vi "portOpen.vi"(3 "COMport":string="COM6") -> (0 "error out":errorcluster)   [LabVIEW 2015]
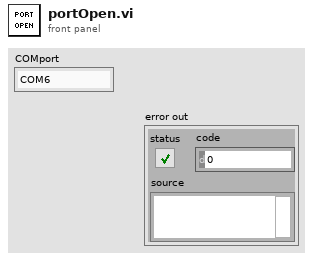
[diagram p1: front panel]
types:
  T1 = cluster{"OpenPort":bool, "ClosePort":bool, "Baudrate":i32, "Wait":u16, "ReadWrite":bool}
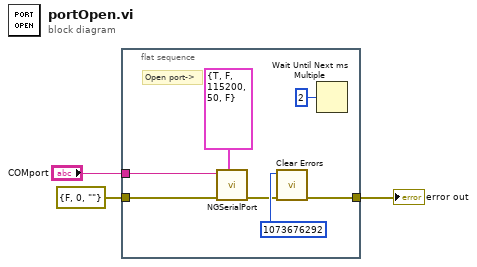
[diagram p0: block diagram]
diagram:
  n1 = flat-sequence {
    tunnel: "COMport" -> [w10]
    tunnel: [w8] -> w2
    tunnel: errorcluster {"status"=FALSE, "code"=0, "source"=""} ("error in") -> [w6]
    frame #0 {
      # "Open port->"
      n2 = call "NGSerialPort.vi"("PortParameters"=T1 {"OpenPort"=TRUE, "ClosePort"=FALSE, "Baudrate"=115200, "Wait"=50, "ReadWrite"=FALSE}, "error in"=w6, "VISA in"=w10) -> ("error out"=w5:errorcluster)  [unwired: 6 in, 2 out]
      n3 = call <vilib>:"Clear Errors.vi"("error in (no error)"=w5, "specific error code to clear (0: all)"=1073676292) -> ("error out"=w8:errorcluster)  [unwired: 4 in, 1 out]
      n4 = Wait Until Next ms Multiple(millisecond multiple=u32 2) -> ()  [unwired: 1 out]
    }
  }
  "error out" <- w2
